vi "Set command-data.vi"(8 "error in (no error)":errorcluster, 9 "Cluster":T1, 10 "Name":string, 11 "Message Response in":refnum<class "Message Response.lvclass">) -> (0 "error out":errorcluster, 3 "Message Response out":refnum<class "Message Response.lvclass">)   [LabVIEW 2016, in "WebSocket Networking.lvlib" / "Message Response.lvclass"]
uses:
  <userlib>/Common Components/WebSocket Networking/Message Response/Message Response.lvclass
  C:/Program Files (x86)/National Instruments/LabVIEW 2016/user.lib/Composed Systems/Stream/Mediator/Classes/Message Interface/Message Interface.lvclass
  <userlib>/Common Components/Common/command-data.ctl
  <userlib>/Common Components/WebSocket Networking/Message Response/Message Response.lvclass/Message Response.ctl
  <userlib>/Composed Systems/Stream/Mediator/Classes/Message Interface/Message Interface.lvclass
  <userlib>/Common Components/Common/Common.lvlib
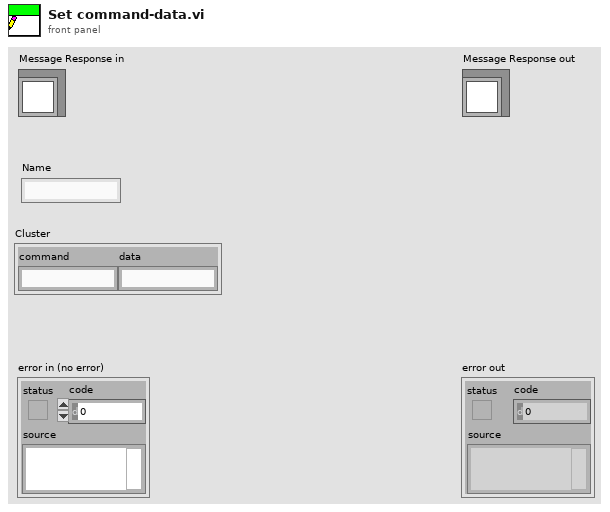
[diagram p1: front panel]
types:
  T1 = typedef "Common.lvlib/command-data.ctl" = cluster{"command":string, "data":string}
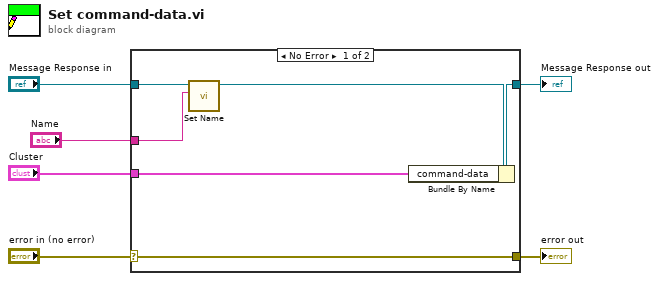
[diagram p0: block diagram]
diagram:
  n1 = case shown="No Error" "error in (no error)" {
    selector: "error in (no error)" -> [w12 w13]
    tunnel: [w12 w13] -> w5
    tunnel: [w11 w14] -> w3
    tunnel: "Message Response in" -> [w9 w14]
    tunnel: "Cluster" -> [w10 _]
    tunnel: "Name" -> [w7 _]
    frame No Error {
      n2 = call <userlib>:"Set Name.vi"("Name"=w7, "Message Interface in"=w9) -> ("Message Interface out"=w8:refnum<class "Message Response.lvclass">)  [unwired: 8 in, 1 out]
      n3 = Bundle By Name(cluster=w8, "command-data"=w10) -> (w11:refnum<class "Message Response.lvclass">)
    }
    frame Error {
    }
  }
  "error out" <- w5
  "Message Response out" <- w3
